vi "8-bit Number to LED.vi"(1 "6-bit Unsigned\n Number (0-63)":u8) -> ()   [LabVIEW 2015]
doc: "This VI accepts an 8-bit unsigned number and outputs it in binary to the sbRIO evaluation board bank of eight LEDs."
uses:
  <vilib>/rvi/eio/common/nirviEmuTemplateMethod_errors.vi
  <vilib>/eio/EIONode/EIONode.xnode
panel:
  # "This VI accepts an 8-bit unsigned number and outputs it in binary to the sbRIO evaluation board bank of six LEDs.  Only the first six binary digits are displayed on the board."
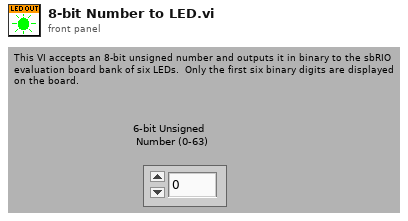
[diagram p1: front panel]
types:
  T1 = cluster{"Boolean array[0]":bool, "Boolean array[1]":bool, "Boolean array[2]":bool, "Boolean array[3]":bool, "Boolean array[4]":bool, "Boolean array[5]":bool, "Boolean array[6]":bool, "Boolean array[7]":bool, "Boolean array[8]":bool}
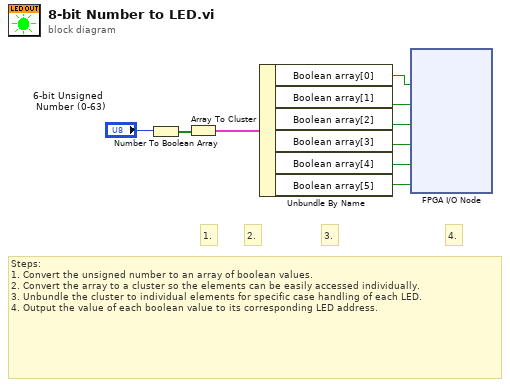
[diagram p0: block diagram]
diagram:
  # "4."
  # "3."
  # "2."
  # "1."
  # "Steps:\n1. Convert the unsigned number to an array of boolean values.\n2. Convert the array to a cluster so the elements can be easily accessed individually.\n3. Unbundle the cluster to individual elements for specific case handling of each LED.\n4. Output the value of each boolean value to its corresponding LED address."
  n1 = Number To Boolean Array(number="6-bit Unsigned\n Number (0-63)") -> (Boolean array=w9:bool[])
  n2 = Array To Cluster(array=w9) -> (cluster=w8:T1)
  n3 = Unbundle By Name(w8) -> ("Boolean array[0]"=w6:bool, "Boolean array[1]"=w5:bool, "Boolean array[2]"=w4:bool, "Boolean array[3]"=w3:bool, "Boolean array[4]"=w2:bool, "Boolean array[5]"=w1:bool)
  n4 = xnode "FPGA I/O Node"("LED 1"=w6, "LED 2"=w5, "LED 3"=w4, "LED 4"=w3, "LED 5"=w2, "LED 6"=w1) -> ()  [unwired: 6 in, 6 out]
